vi "INIT STOP.vi"(4 "error in (no error)":errorcluster) -> (1 "error out":errorcluster)   [LabVIEW 2013, in "GlobalStop(dev).lvlib"]
uses:
  GlobalStop(dev).lvlib
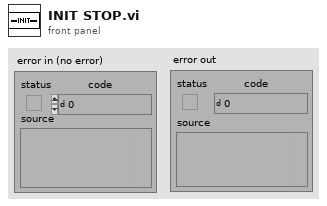
[diagram p1: front panel]
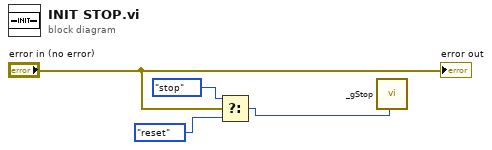
[diagram p0: block diagram]
diagram:
  n1 = Select(t=enum16{"reset", "get", "stop"}."stop" ("op"), s="error in (no error)", f=enum16{"reset", "get", "stop"}."reset" ("op")) -> (s? t:f=w2:enum16{"reset", "get", "stop"})
  n2 = call "_gStop.vi"("op"=w2) -> ()  [unwired: 10 in, 1 out]
  "error out" <- "error in (no error)"
